vi "Destroy.vi"(8 "error in (no error)":errorcluster, 11 "Agilent DSO-X 3032A in":refnum<class "Agilent DSO-X 3032A.lvclass">) -> (3 "Agilent DSO-X 3032A out":refnum<class "Agilent DSO-X 3032A.lvclass">)   [LabVIEW 2014, in "Agilent DSO-X 3032A.lvclass"]
uses:
  Agilent DSO-X 3032A.lvclass
  Agilent DSO-X 3032A.lvclass/Agilent DSO-X 3032A.ctl
  Framework/Hardware/ReadoutDevice/ReadoutDevice.lvclass
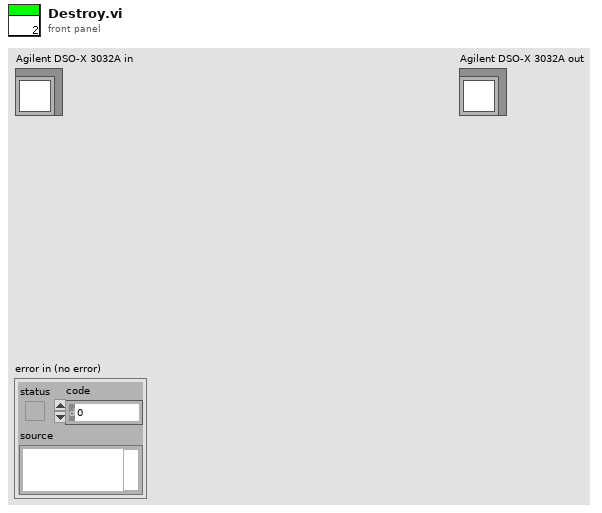
[diagram p1: front panel]
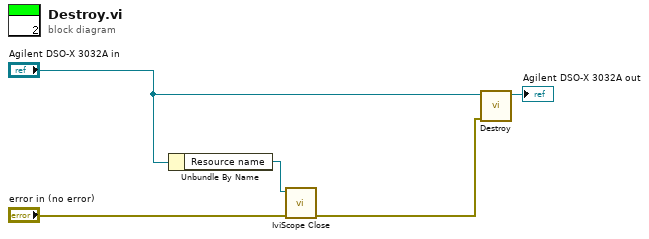
[diagram p0: block diagram]
diagram:
  n1 = Unbundle By Name("Agilent DSO-X 3032A in") -> ("Resource name"=w1:refnum<k15>)
  n2 = call <vilib>:"IviScope Close.vi"("error in (no error)"="error in (no error)", "instrument handle"=w1) -> ("error out"=w2:errorcluster)  [unwired: 9 out]
  n3 = call-parent "Destroy.vi"("error in (no error)"=w2, "Device in"="Agilent DSO-X 3032A in") -> ("Device out"=→"Agilent DSO-X 3032A out":refnum<class "Agilent DSO-X 3032A.lvclass">)  [unwired: 9 in]
